vi "InitDelays.vi"(11 "config in":T1) -> (3 "config out":T1)   [LabVIEW 2017, in "TrendAlarm.lvlib"]
uses:
  <vilib>/addons/InsightCM/Devices/Shared/Common/TrendAlarm/TrendAlarm.lvlib
  <vilib>/addons/InsightCM/Devices/Shared/Common/TrendAlarm/controls/config.ctl
  <vilib>/addons/InsightCM/Devices/Shared/Common/TrendAlarm/controls/TransitionCache.ctl
  <vilib>/addons/InsightCM/MessageBus/Base/controls/TrendAlarmTransition.ctl
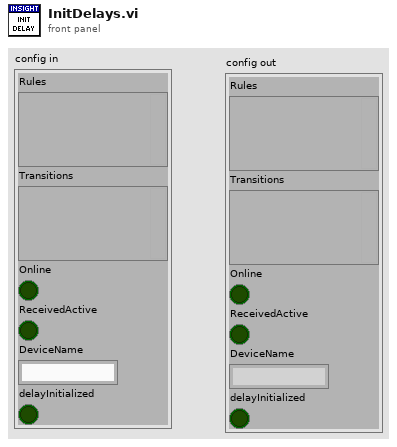
[diagram p1: front panel]
types:
  T1 = typedef "TrendAlarm.lvlib/config.ctl" = cluster{"Rules":variant, "Transitions":variant, "Online":bool, "ReceivedActive":bool, "DeviceName":string, "delayInitialized":bool}
  T2 = typedef "TrendAlarm.lvlib/TransitionCache.ctl" = cluster{"RuleId":string, "MaxSeverity":i32, "LastTransition":T3, "OnTime":timestamp, "OffTime":timestamp}
  T3 = typedef "TrendAlarmTransition.ctl" = cluster{"At":i64, "Severity":i32, "Value":dbl}
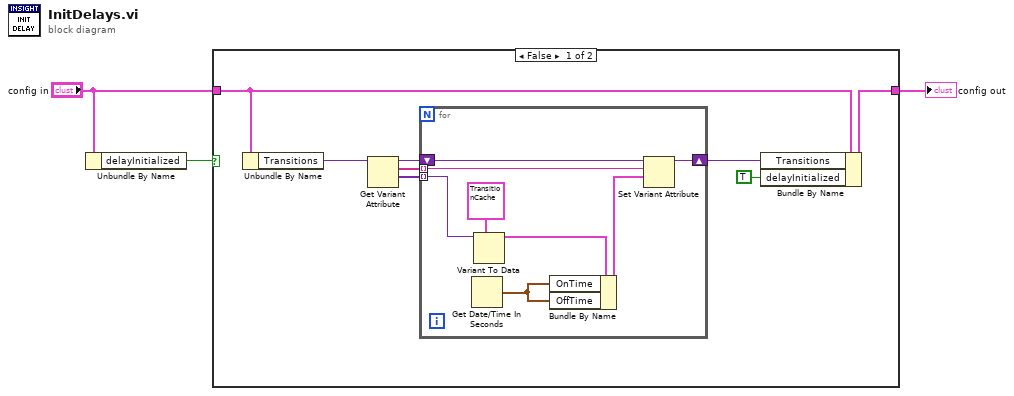
[diagram p0: block diagram]
diagram:
  n1 = Unbundle By Name("config in") -> ("delayInitialized"=w3:bool)
  n2 = case shown="False" w3 {
    tunnel: "config in" -> [w7 w20]
    tunnel: [w5 w20] -> w1
    frame False {
      n3 = Unbundle By Name(w7) -> ("Transitions"=w11:variant)
      n4 = Get Variant Attribute(Variant=w11) -> (duplicate Variant=w10:variant, names=w9:string[], values=w8:variant[])  [unwired: 3 in, 1 out]
      n5 = for {
        shift-right: [w18] -> w6
        shift-left: w10 -> [w19]
        tunnel: w9 -> [w16] mode=indexing
        tunnel: w8 -> [w15] mode=indexing
        n6 = Get Date/Time In Seconds() -> (seconds since 1Jan1904=w12:timestamp)
        n7 = Variant To Data(type=T2 {"RuleId"="", "MaxSeverity"=0, "LastTransition"={"At"=0, "Severity"=0, "Value"=0.0}, "OnTime"=timestamp(0 s since 1904-01-01), "OffTime"=timestamp(0 s since 1904-01-01)} ("TransitionCache"), Variant=w15) -> (data=w13:T2)  [unwired: 1 in, 1 out]
        n8 = Bundle By Name(cluster=w13, "OnTime"=w12, "OffTime"=w12) -> (w17:T2)
        n9 = Set Variant Attribute(Variant=w19, name=w16, value=w17) -> (Variant out=w18:variant)  [unwired: 1 in, 2 out]
      }
      n10 = Bundle By Name(cluster=w7, "Transitions"=w6, "delayInitialized"=TRUE) -> (w5:T1)
    }
    frame True {
    }
  }
  "config out" <- w1
